vi "detector de tapa.vi"() -> ()   [LabVIEW 2020]
uses:
  <vilib>/userDefined/High Color/IMAQdx.ctl
  <vilib>/vision/Management.llb/Cast Image 2 Method.ctl
  <vilib>/vision/driver/NI_Vision_Acquisition_Software.lvlib
  <vilib>/vision/NI_Vision_Development_Module.lvlib
panel:
  out "Angle":sgl
  out "y":sgl
  out "x":sgl
  out "tapa detectada":bool
  out "Number of Matches":i32
  out "Rectangle":T1 {"Rotation" min=-90.0 max=90.0 step=1.0 format="%.2f"; "Left" scale=0.0..1024.0; "Right" scale=0.0..1024.0}
  out "Matches (real-world)":T2(array[cluster]) {"Bounding Box"."y" format="%.2f"; "Bounding Box"."x" format="%.2f"; "Score" format="%.2f"; "Scale" format="%.2f"; "Angle" format="%.2f"; "Position"."y" format="%.2f"; "Position"."x" format="%.2f"}
  out "Image 4":T3(plugin-control)
  out "patron":T3(plugin-control)
  in  "File Path":path
  out "Image 3":T3(plugin-control)
  out "Image 2":T3(plugin-control)
  in  "Session In":T4="cam1"
  in  "stop":bool
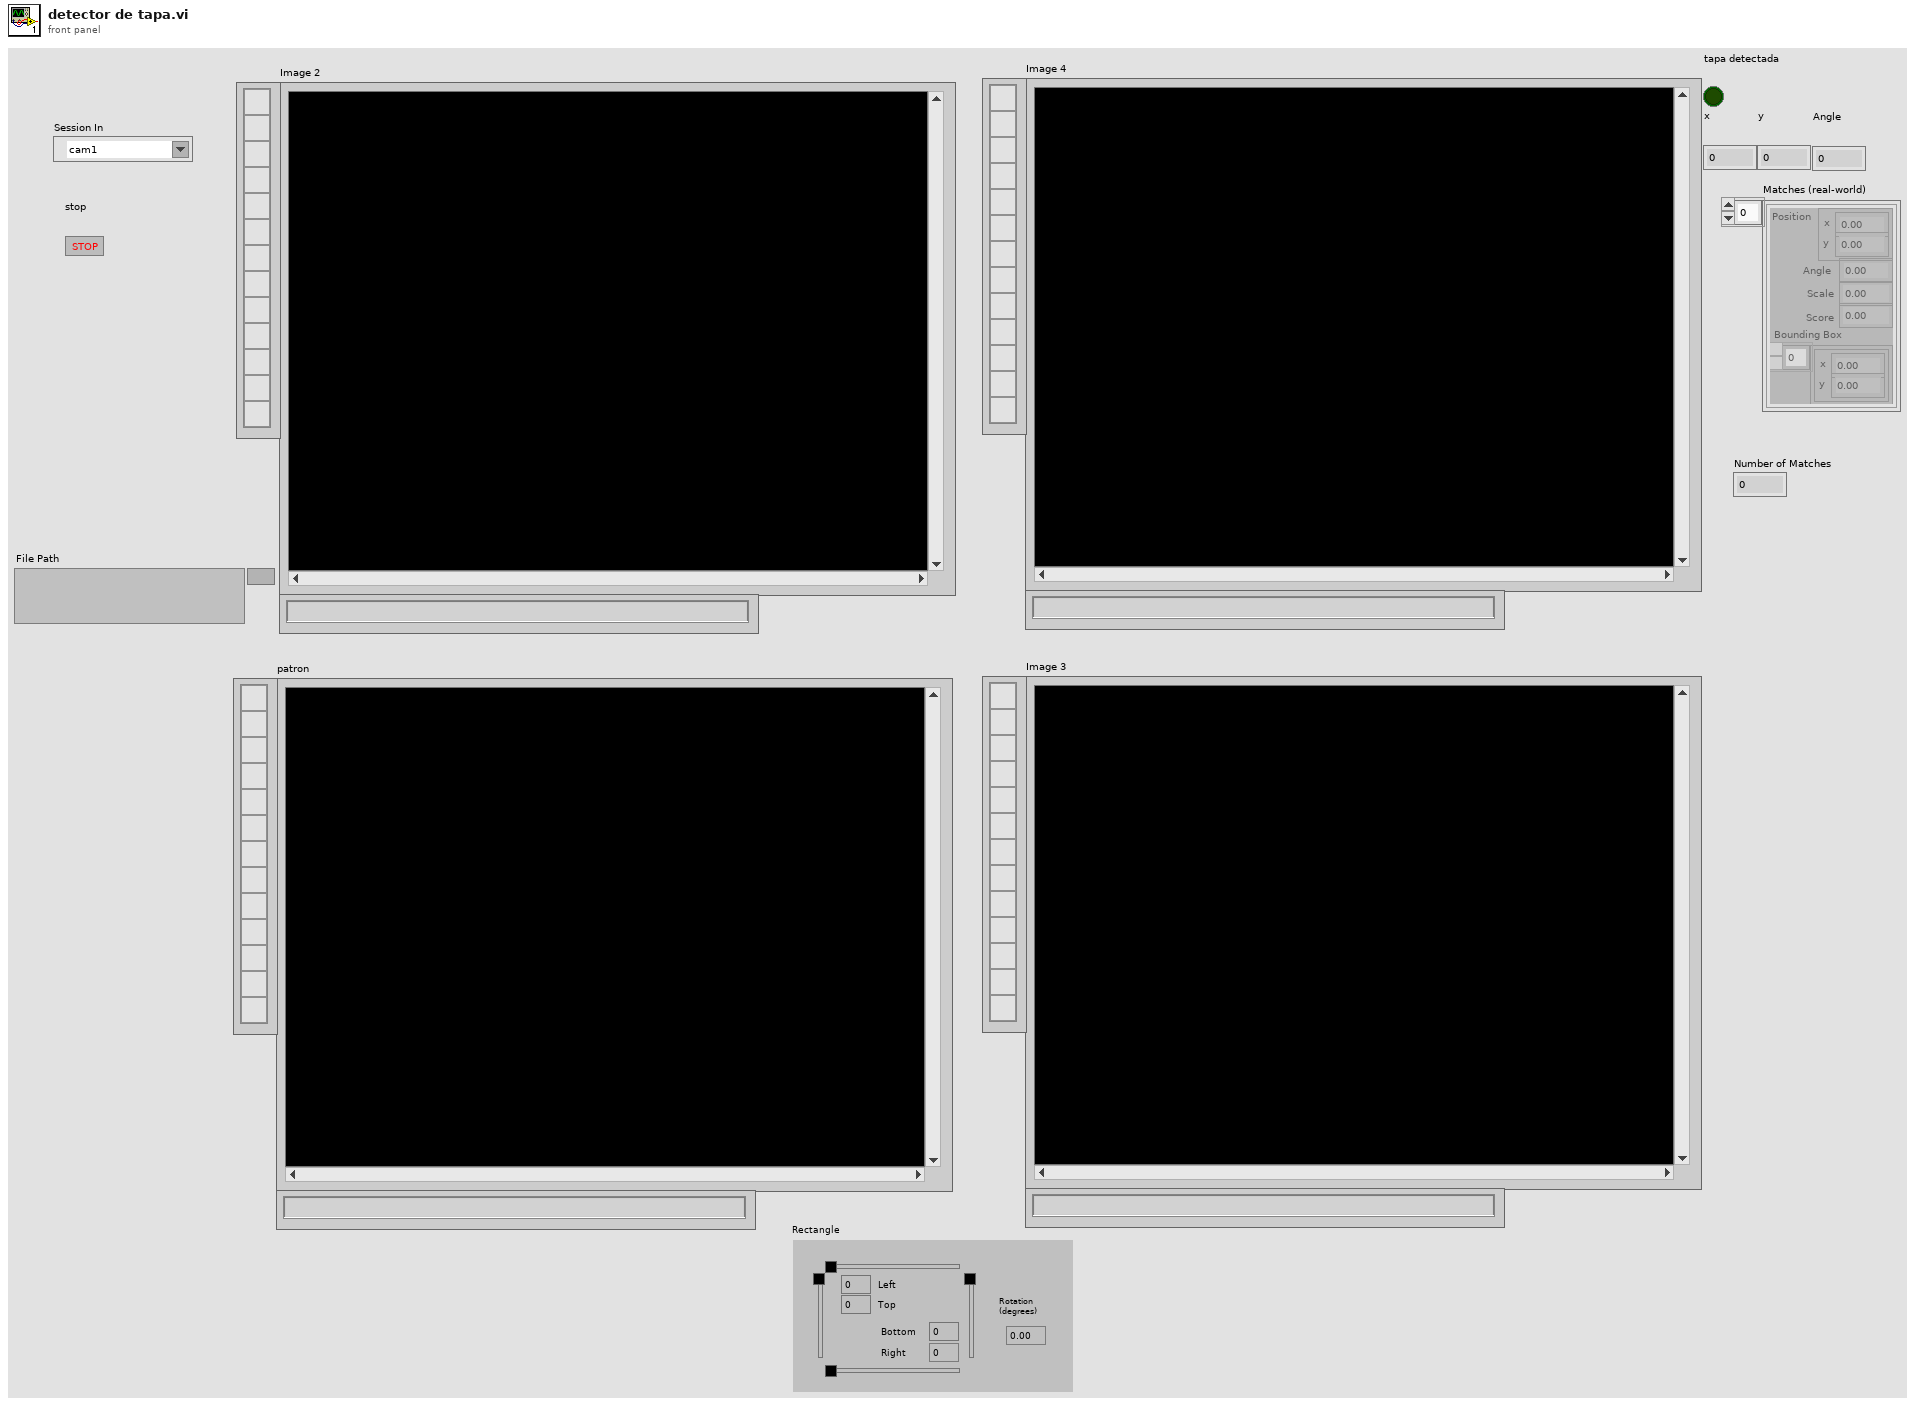
[diagram p1: front panel]
types:
  T1 = typedef "IMAQ Rectangle" = cluster{"Left":i32, "Top":i32, "Right":i32, "Bottom":i32, "Rotation":dbl}
  T2 = cluster{"Position":cluster{"x":sgl, "y":sgl}, "Angle":sgl, "Scale":sgl, "Score":sgl, "Bounding Box":cluster{"x":sgl, "y":sgl}[]}[]
  T3 = typedef "IMAQ Image.ctl" = refnum<image>
  T4 = typedef "IMAQdx.ctl" = refnum<k21>
  T5 = cluster{"Number of Matches Requested":i32, "Minimum Match Score":sgl, "Angle Ranges":cluster{"Start Angle":sgl, "End Angle":sgl}[]}
  T6 = typedef "Image Type" = u32
  T7 = typedef "Cast Image 2 Method.ctl" = u32
  T8 = cluster{"Global Rectangle":i32[], "Contours":cluster{"Contour Type":u32, "ROI Type":u32, "Points":i32[]}[]}
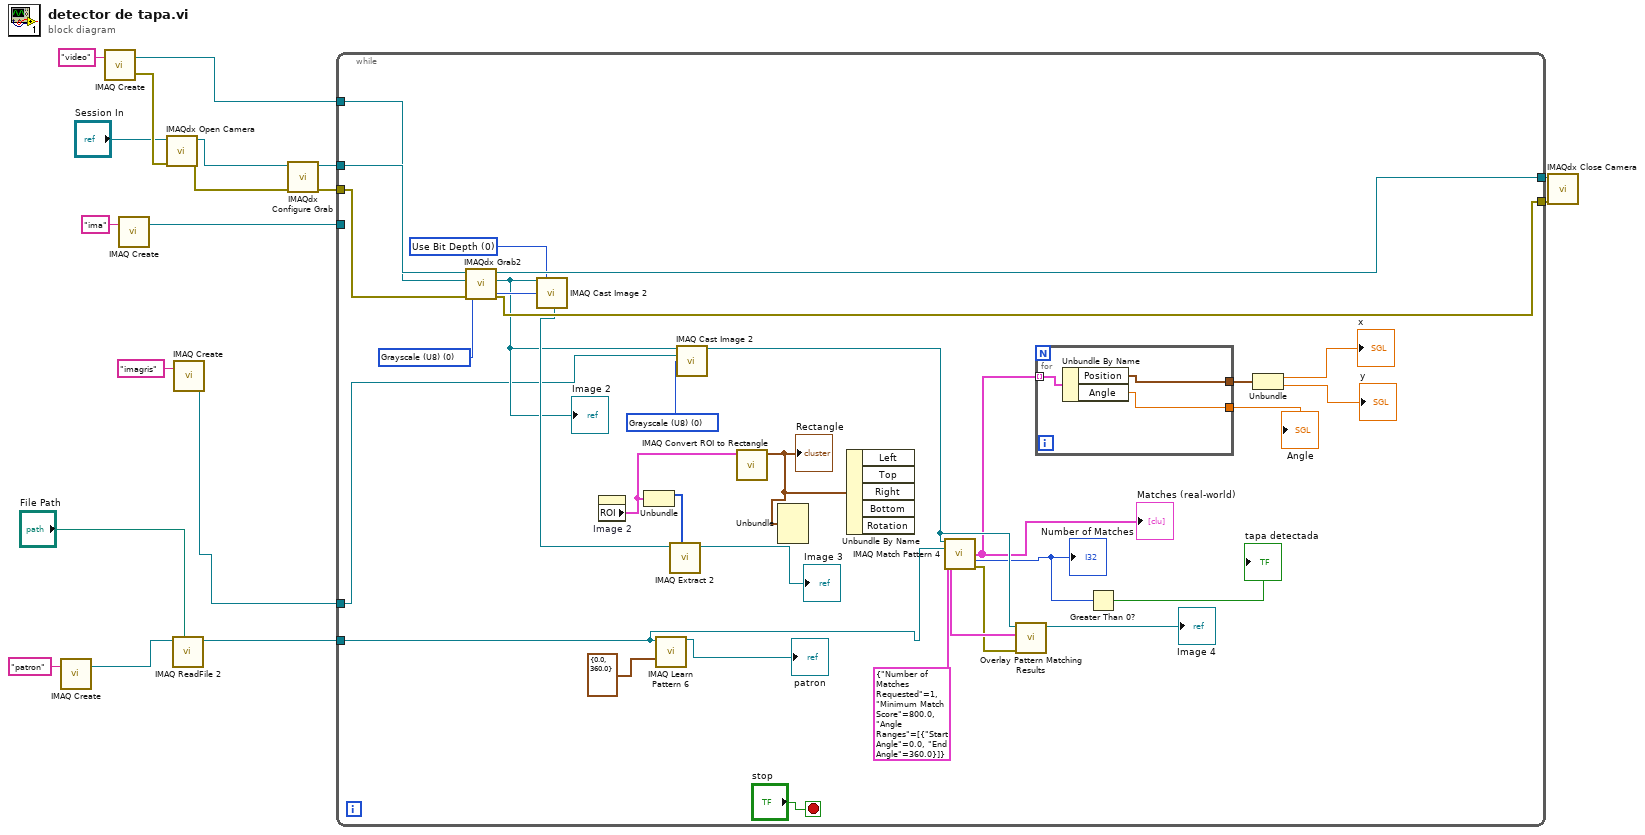
[diagram p0: block diagram]
diagram:
  n1 = call "IMAQ Create"("Image Name"="patron") -> ("New Image"=w2:T3)  [unwired: 4 in, 1 out]
  n2 = call "IMAQ Create"("Image Name"="video") -> ("New Image"=w15:T3, "error out"=w18:errorcluster)  [unwired: 4 in]
  n3 = call "IMAQ Create"("Image Name"="ima") -> ("New Image"=w7:T3)  [unwired: 4 in, 1 out]
  n4 = call <vilib>:"IMAQdx Open Camera.vi"("error in"=w18, "Session In"="Session In") -> ("error out"=w11:errorcluster, "Session Out"=w17:T4)  [unwired: 8 in]
  n5 = call "IMAQ ReadFile 2"("File Path"="File Path", "Image"=w2) -> ("Image Out"=w1:T3)  [unwired: 5 in, 4 out]
  n6 = call "IMAQ Create"("Image Name"="imagris") -> ("New Image"=w5:T3)  [unwired: 4 in, 1 out]
  n7 = call <vilib>:"IMAQdx Configure Grab.vi"("error in"=w11, "Session In"=w17) -> ("error out"=w12:errorcluster, "Session Out"=w16:T4)  [unwired: 8 in]
  n8 = while {
    tunnel: w16 -> [w49]
    tunnel: w15 -> [w48]
    tunnel: [w45] -> w14
    tunnel: [w44] -> w13
    tunnel: w12 -> [w46]
    tunnel: w7 -> [_]
    tunnel: w5 -> [w30]
    tunnel: w1 -> [w36]
    stop <- "stop" stop-if-true
    w31 = T6 0 items=["Grayscale (U8)", "Grayscale (I16)", "Grayscale (SGL)", "Complex (CSG)", "RGB (U32)", "HSL (U32)", "RGB (U64)", "Grayscale (U16)"] ("Image Type")
    w40 = T6 0 items=["Grayscale (U8)", "Grayscale (I16)", "Grayscale (SGL)", "Complex (CSG)", "RGB (U32)", "HSL (U32)", "RGB (U64)", "Grayscale (U16)"] ("Image Type")
    w43 = T7 0 items=["Use Bit Depth", "Shift", "Use Lookup Table"] ("Method")
    n9 = call <vilib>:"IMAQdx Grab2.vi"("error in"=w46, "Image In"=w48, "Session In"=w49) -> ("error out"=w44:errorcluster, "Image Out"=w33:T3, "Session Out"=w45:T4)  [unwired: 5 in, 1 out]
    "Image 2" <- w33
    n10 = call "IMAQ Cast Image 2"("Image Src"=w33, "Method"=w43, "Image Type"=w40) -> ("Image Dst Out"=w34:T3)  [unwired: 11 in, 1 out]
    n11 = property on="Image 2" class="ImageControl"() -> ("ROI"=w28:T8)  [unwired: 2 in, 2 out]
    n12 = Unbundle(w28) -> ("Global Rectangle"=w42:i32[])  [unwired: 1 out]
    n13 = call "IMAQ Learn Pattern 6"("Image"=w36, "Angle Range"=cluster{"Start Angle":sgl, "End Angle":sgl} {"Start Angle"=0.0, "End Angle"=360.0}) -> ("Template Image Out"=→"patron":T3)  [unwired: 11 in, 2 out]
    n14 = call "IMAQ Extract 2"("Optional Rectangle"=w42, "Image Src"=w34) -> ("Image Dst Out"=→"Image 3":T3)  [unwired: 8 in, 1 out]
    n15 = call "IMAQ Cast Image 2"("Image Src"=w33, "Image Dst"=w30, "Image Type"=w31) -> ("Image Dst Out"=w32:T3)  [unwired: 11 in, 1 out]
    n16 = call "IMAQ Convert ROI to Rectangle"("ROI Descriptor"=w28) -> ("Rectangle"=w22:T1)  [unwired: 8 in, 1 out]
    "Rectangle" <- w22
    n17 = Unbundle(w22) -> ()  [unwired: 5 out]
    n18 = Unbundle By Name(w22) -> ()  [unwired: 5 out]
    n19 = call "IMAQ Match Pattern 4"("Image"=w32, "Template Image"=w36, "Parameters"=T5 {"Number of Matches Requested"=1, "Minimum Match Score"=800.0, "Angle Ranges"=[{"Start Angle"=0.0, "End Angle"=360.0}]}) -> ("Matches (pixel)"=w38:T2, "Matches (real-world)"=w29:T2, "Number of Matches"=w26:i32, "error out"=w37:errorcluster)  [unwired: 8 in, 1 out]
    "Matches (real-world)" <- w29
    "Number of Matches" <- w26
    n20 = call "Overlay Pattern Matching Results.vi"("error in"=w37, "Matches"=w38, "Image"=w32) -> ("Image Out"=→"Image 4":T3)  [unwired: 7 in, 1 out]
    n21 = for {
      tunnel: w29 -> [w52] mode=indexing
      tunnel: [w51] -> w27
      tunnel: [w50] -> w21
      n22 = Unbundle By Name(w52) -> ("Position"=w51:cluster{"x":sgl, "y":sgl}, "Angle"=w50:sgl)
    }
    "Angle" <- w21
    n23 = Greater Than 0?(x=w26) -> (x > 0?=→"tapa detectada":bool)
    n24 = Unbundle(w27) -> ("x"=→"x":sgl, "y"=→"y":sgl)
  }
  n25 = call <vilib>:"IMAQdx Close Camera.vi"("error in"=w13, "Session In"=w14) -> ()  [unwired: 9 in, 1 out]
